vi "Valid Resource.vi"(8 "error in (no error)":errorcluster, 10 "RP2040.lvlib:VisaResource":refnum<class "VisaResource.lvclass">) -> (0 "error out":errorcluster, 2 "Valid?":bool)   [LabVIEW 2020, in "RP2040.lvlib" / "RP2040Target.lvclass"]
uses:
  RP2040Target.lvclass
  VisaResource/VisaResource.lvclass
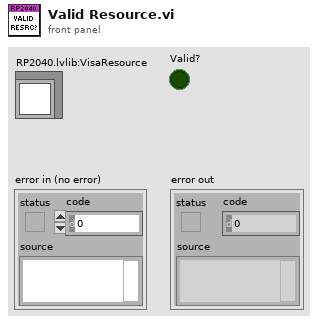
[diagram p1: front panel]
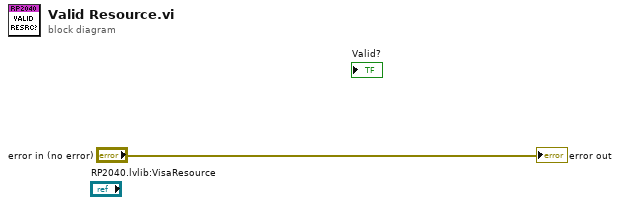
[diagram p0: block diagram]
diagram:
  "error out" <- "error in (no error)"
